vi "crop_image.vi"(8 "bboxes":T1(array[cluster]), 9 "classes":string[](array[string]), 10 "Dataset path":path, 11 "Image path":path) -> ()   [LabVIEW 2024]
uses:
  <vilib>/vision/NI_Vision_Development_Module.lvlib
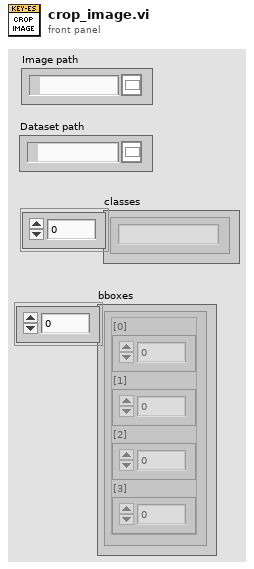
[diagram p1: front panel]
types:
  T1 = cluster{"[0]":i32, "[1]":i32, "[2]":i32, "[3]":i32}[]
  T2 = typedef "Image Type" = u32
  T3 = typedef "IMAQ Image.ctl" = refnum<image>
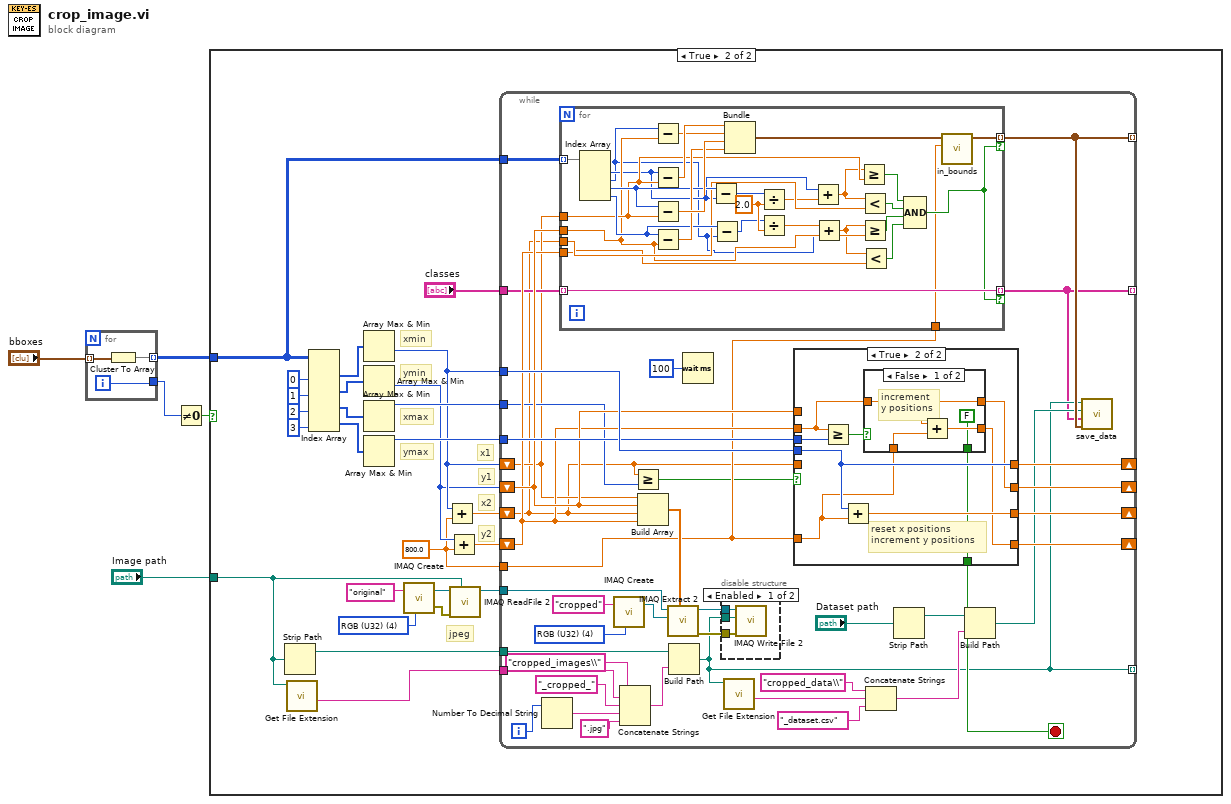
[diagram p0: block diagram]
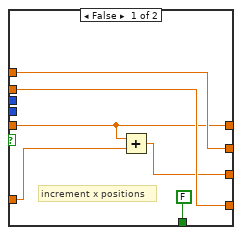
[diagram p4: hidden frame]
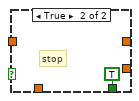
[diagram p5: hidden frame]
diagram:
  n1 = for {
    tunnel: "bboxes" -> [w8] mode=indexing
    tunnel: [w7] -> w3 mode=indexing
    tunnel: [w6] -> w1
    i -> [w6]
    n2 = Cluster To Array(cluster=w8) -> (array=w7:i32[])
  }
  n3 = Not Equal To 0?(x=w1) -> (x != 0?=w2:bool)
  n4 = case shown="True" w2 {
    tunnel: "Image path" -> [_ w12]
    tunnel: w3 -> [_ w10]
    frame False {
    }
    frame True {
      w15 = T2 4 items=["Grayscale (U8)", "Grayscale (I16)", "Grayscale (SGL)", "Complex (CSG)", "RGB (U32)", "HSL (U32)", "RGB (U64)", "Grayscale (U16)"] ("Image Type")
      w11 = 800.0 ("y")
      # "jpeg"
      # "y1"
      # "x1"
      # "y2"
      # "x2"
      # "ymax"
      # "xmax"
      # "ymin"
      # "xmin"
      n5 = Strip Path(path=w12) -> (stripped path=w21:path)  [unwired: 1 out]
      n6 = call <vilib>:"Get File Extension.vi"("file"=w12) -> ("filename without extension"=w20:string)  [unwired: 6 in, 4 out]
      n7 = Index Array(array=w10, index (col) #1=0 ("disabled index (col)"), index (col) #2=1 ("index (col)"), index (col) #3=2 ("index (col)"), index (col) #4=3 ("index (col)")) -> (element #1=w29:i32[], element #2=w28:i32[], element #3=w27:i32[], element #4=w26:i32[])  [unwired: 4 in]
      n8 = Array Max & Min(array=w29) -> (min value=w19:i32)  [unwired: 3 out]
      n9 = Array Max & Min(array=w28) -> (min value=w18:i32)  [unwired: 3 out]
      n10 = Array Max & Min(array=w27) -> (max value=w25:i32)  [unwired: 3 out]
      n11 = Array Max & Min(array=w26) -> (max value=w24:i32)  [unwired: 3 out]
      n12 = call "IMAQ Create"("Image Name"="original", "Image Type"=w15) -> ("New Image"=w17:T3, "error out"=w14:errorcluster)  [unwired: 3 in]
      n13 = Add(x=w19, y=w11) -> (x+y=w23:dbl)
      n14 = Add(x=w18, y=w11) -> (x+y=w22:dbl)
      n15 = call "IMAQ ReadFile 2"("File Path"=w12, "error in (no error)"=w14, "Image"=w17) -> ("Image Out"=w13:T3)  [unwired: 4 in, 4 out]
      n16 = while {
        tunnel: w19 -> [w67]
        tunnel: w25 -> [w38]
        tunnel: w24 -> [w62]
        tunnel: w21 -> [w68]
        tunnel: w20 -> [w69]
        shift-right: [w65] -> _
        shift-left: w23 -> [w35]
        shift-right: [w64] -> _
        shift-left: w22 -> [w54]
        shift-right: [w66] -> _
        shift-left: w19 -> [w36]
        shift-right: [w63] -> _
        shift-left: w18 -> [w55]
        tunnel: w13 -> [w57]
        tunnel: w11 -> [w43]
        tunnel: w10 -> [w56]
        tunnel: "classes" -> [w53]
        tunnel: [w46] -> _ mode=indexing
        tunnel: [w37] -> _ mode=indexing
        tunnel: [w44] -> _ mode=indexing
        i -> [w74]
        stop <- w61 stop-if-true
        w59 = T2 4 items=["Grayscale (U8)", "Grayscale (I16)", "Grayscale (SGL)", "Complex (CSG)", "RGB (U32)", "HSL (U32)", "RGB (U64)", "Grayscale (U16)"] ("Image Type")
        n17 = Number To Decimal String(number=w74) -> (decimal integer string=w72:string)  [unwired: 1 in]
        n18 = for {
          tunnel: w56 -> [w107] mode=indexing
          tunnel: w36 -> [w92]
          tunnel: w55 -> [w89]
          tunnel: w54 -> [w90]
          tunnel: w35 -> [w91]
          tunnel: [w80] -> w46 mode=indexing if=w82
          tunnel: w53 -> [w106] mode=indexing
          tunnel: [w106] -> w37 mode=indexing if=w82
          tunnel: w43 -> [w79]
          w101 = 2.0 ("y")
          n19 = Index Array(array=w107) -> (element #1=w86:i32, element #2=w85:i32, element #3=w100:i32, element #4=w99:i32)  [unwired: 4 in]
          n20 = Subtract(x=w85, y=w89) -> (x-y=w104:dbl)
          n21 = Subtract(x=w86, y=w92) -> (x-y=w105:dbl)
          n22 = Subtract(x=w100, y=w92) -> (x-y=w103:dbl)
          n23 = Subtract(x=w99, y=w89) -> (x-y=w102:dbl)
          n24 = Subtract(x=w100, y=w86) -> (x-y=w98:i32)
          n25 = Subtract(x=w99, y=w85) -> (x-y=w97:i32)
          n26 = Bundle(w105, w104, w103, w102) -> (w81:cluster{dbl, dbl, dbl, dbl})  [unwired: 1 in]
          n27 = Divide(x=w98, y=w101) -> (x/y=w88:dbl)
          n28 = Divide(x=w97, y=w101) -> (x/y=w87:dbl)
          n29 = Add(x=w86, y=w88) -> (x+y=w84:dbl)
          n30 = Add(x=w87, y=w85) -> (x+y=w83:dbl)
          n31 = Greater Or Equal?(x=w84, y=w92) -> (x >= y?=w96:bool)
          n32 = Less?(x=w84, y=w91) -> (x < y?=w93:bool)
          n33 = Greater Or Equal?(x=w83, y=w89) -> (x >= y?=w94:bool)
          n34 = Less?(x=w83, y=w90) -> (x < y?=w95:bool)
          n35 = Compound Arithmetic op=AND(w96, w93, w94, w95) -> (w82:bool)
          n36 = call "in_bounds.vi"("size"=w79, "bbox"=w81) -> ("bbox_out"=w80:cluster{"y":dbl, "y":dbl, "y":dbl, "y":dbl})  [unwired: 9 in]
        }
        n37 = call "IMAQ Create"("Image Name"="cropped", "Image Type"=w59) -> ("New Image"=w58:T3)  [unwired: 3 in, 1 out]
        n38 = Concatenate Strings("cropped_images\\" ("name or relative path"), w69, "_cropped_" ("name or relative path"), w72, ".jpg" ("string")) -> (w70:string)
        n39 = Greater Or Equal?(x=w35, y=w38) -> (x >= y?=w39:bool)
        n40 = Build Array(w36, w55, w35, w54) -> (w52:dbl[])
        n41 = call "IMAQ Extract 2"("Optional Rectangle"=w52, "Image Dst"=w58, "Image Src"=w57) -> ("error out"=w75:errorcluster, "Image Dst Out"=w51:T3)  [unwired: 7 in]
        n42 = Build Path(base path=w68, name or relative path=w70) -> (appended path=w44:path)
        n43 = Wait (ms)(milliseconds to wait=u32 100) -> ()  [unwired: 1 out]
        n44 = disable-structure shown="Enabled" {
          disable-tunnel: w51 -> [w78 _]
          disable-tunnel: w75 -> [w77 _]
          disable-tunnel: w44 -> [w76 _]
          frame Enabled {
            n45 = call-poly "IMAQ Write File 2"("error in (no error)"=w77, "File Path"=w76, "Image"=w78) -> ()  [unwired: 7 in, 2 out]
          }
          frame Disabled {
          }
        }
        n46 = call <vilib>:"Get File Extension.vi"("file"=w44) -> ("filename without extension"=w49:string)  [unwired: 6 in, 4 out]
        n47 = case shown="True" w39 {
          tunnel: w67 -> [_ w121]
          tunnel: [w110 w121] -> w66
          tunnel: [w109 w122] -> w65
          tunnel: [w112 w117] -> w64
          tunnel: [w111 w118] -> w63
          tunnel: w54 -> [w112 w114]
          tunnel: w62 -> [_ w120]
          tunnel: [FALSE w116] -> w61
          tunnel: w55 -> [w111 _]
          tunnel: w35 -> [w110 _]
          tunnel: w43 -> [w108 w115]
          frame False {
            # "increment x positions"
            n48 = Add(x=w110, y=w108) -> (x+y=w109:dbl)
          }
          frame True {
            # "reset x positions\nincrement y positions"
            n49 = Greater Or Equal?(x=w114, y=w120) -> (x >= y?=w119:bool)
            n50 = Add(x=w121, y=w115) -> (x+y=w122:dbl)
            n51 = case shown="False" w119 {
              tunnel: [w126 _] -> w118
              tunnel: [w125 _] -> w117
              tunnel: w114 -> [w126 _]
              tunnel: [FALSE TRUE] -> w116
              tunnel: w115 -> [w123 _]
              frame False {
                # "increment\ny positions"
                n52 = Add(x=w126, y=w123) -> (x+y=w125:dbl)
              }
              frame True {
                # "stop"
              }
            }
          }
        }
        n53 = Concatenate Strings("cropped_data\\" ("name or relative path"), w49, "_dataset.csv" ("name or relative path")) -> (w47:string)
        n54 = Strip Path(path="Dataset path") -> (stripped path=w34:path)  [unwired: 1 out]
        n55 = Build Path(base path=w34, name or relative path=w47) -> (appended path=w45:path)
        n56 = call "save_data.vi"("bboxes"=w46, "classes"=w37, "Dataset path"=w45, "Image path"=w44) -> ()  [unwired: 8 in]
      }
    }
  }
